vi "inFrontBall.vi"(4 "DistanceAttackerToBackBall":dbl, 6 "Target":dbl[](array[numeric]), 8 "error in (no error)":errorcluster, 9 "Pos_est adapted":dbl[](array[numeric]), 10 "BallPos":dbl[](array[numeric]), 11 "KickToSkill in":refnum<class "KickToSkill.lvclass">) -> (0 "error out":errorcluster, 2 "FrontBallPos":dbl[](array[numeric]), 3 "KickToSkill out":refnum<class "KickToSkill.lvclass">)   [LabVIEW 2023, in "KickToSkill.lvclass"]
uses:
  KickToSkill.lvclass
  <vilib>/Analysis/_algsub.llb/Real Vector Norm.vi
  KickToSkill.lvclass/KickToSkill.ctl
  <vilib>/Analysis/NI_AALPro.lvlib
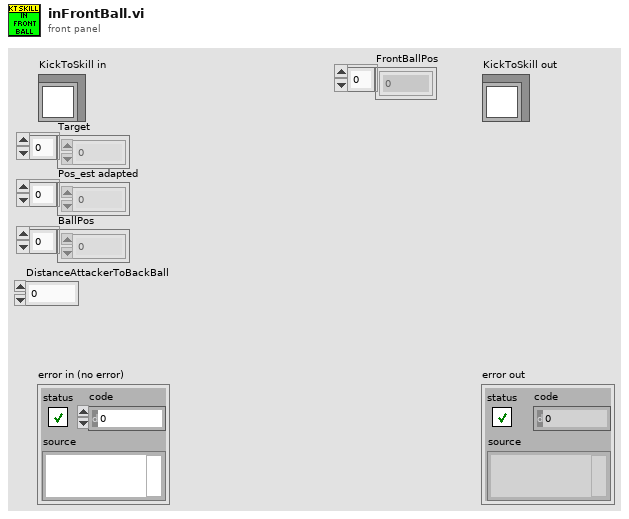
[diagram p1: front panel]
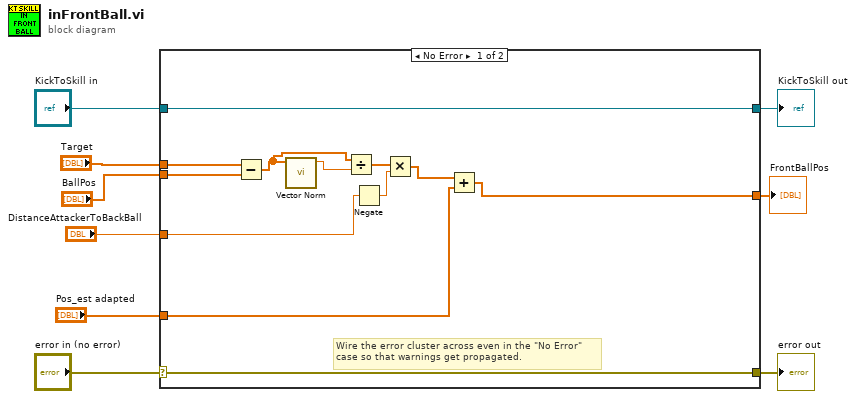
[diagram p0: block diagram]
diagram:
  n1 = case shown="No Error" "error in (no error)" {
    selector: "error in (no error)" -> [w20 w23]
    tunnel: [w20 w23] -> w8
    tunnel: [w21 w22] -> w6
    tunnel: "KickToSkill in" -> [w21 w22]
    tunnel: "Target" -> [w19 _]
    tunnel: "BallPos" -> [w18 _]
    tunnel: "Pos_est adapted" -> [w13 _]
    tunnel: [w12 _] -> w2
    tunnel: "DistanceAttackerToBackBall" -> [w11 _]
    frame No Error {
      # "Wire the error cluster across even in the \"No Error\"\ncase so that warnings get propagated."
      n2 = Subtract(x=w19, y=w18) -> (x-y=w17:dbl[])
      n3 = call-poly <vilib>:"Vector Norm.vi"("Input Vector"=w17) -> ("norm"=w16:dbl)  [unwired: 9 in, 1 out]
      n4 = Divide(x=w17, y=w16) -> (x/y=w15:dbl[])
      n5 = Negate(x=w11) -> (-x=w10:dbl)
      n6 = Multiply(x=w15, y=w10) -> (x*y=w14:dbl[])
      n7 = Add(x=w14, y=w13) -> (x+y=w12:dbl[])
    }
    frame Error {
    }
  }
  "error out" <- w8
  "KickToSkill out" <- w6
  "FrontBallPos" <- w2
